vi "HEWH RLT PRAT.vi"() -> ()   [LabVIEW 2016] (continued)
        n1090 = Unbundle By Name(w2500) -> ("Plot Array C"=w2502:dbl[][], "C Data Array"=w2497:string[][], "File Locations C.New Summary Created"=w2498:bool, "Core HEWH Data Input C.LV Program"=w2491:T24)
        n1091 = case shown="\"PRAT\", \"HEWH RLT\"" w2491 {
          tunnel: [TRUE ("Reset After 24hrs") FALSE ("Reset After 24hrs")] -> w2490
          frame Default {
          }
          frame "PRAT", "HEWH RLT" {
          }
        }
        n1092 = Transpose 2D Array(2D array=w2497) -> (transposed array=w2496:string[][])
        n1093 = call <vilib>:"Add State(s) to Queue__jki_lib_state_machine.vi"("State(s) in (\"\")"=w2510) -> ("States Out"=w2509:string)  [unwired: 14 in]
        n1094 = call "UTILITY MultiPlot.vi"("Y-Axis-2"="Y-Axis2 - Station C", "Y-Axis-1"="Y-Axis1 - Station C", "X-Axis"="X-Axis - Station C", "Save Data"=w2496, "Plot Array"=w2502) -> ("Plot Cluster"=w2507:T34)  [unwired: 5 in, 1 out]
        n1095 = call "UTILITY Create Plot Array.vi"("Save Data"=w2496, "Plot Array in"=w2502) -> ("Plot Array out"=w2495:dbl[][])  [unwired: 8 in, 1 out]
        n1096 = call "UTILITY Array Reset.vi"("Reset After 24hrs"=w2490, "Plot Array Input"=w2495) -> ("Reset Array"=w2494:bool)  [unwired: 9 in]
        n1097 = case shown="False" "Pause Graph C" {
          tunnel: w2507 -> [w2517 _]
          tunnel: "X-Axis - Station C" -> [w2516 _]
          tunnel: "Y-Axis1 - Station C" -> [w2515 _]
          frame False {
            n1098 = property on="XY Graph - Station C" class="XYGraph (strict)"("XScale.NameLbl.Text"=w2516, "YScale.NameLbl.Text"=w2515) -> ()  [unwired: 2 in, 2 out]
            "XY Graph - Station C" <- w2517
          }
          frame True {
          }
        }
        n1099 = Compound Arithmetic op=OR("Clear Graph Data C", w2498, w2494) -> (w2503:bool)
        n1100 = case shown="False" w2503 {
          tunnel: w2495 -> [w2513 _]
          tunnel: [w2513 dbl[][] [] ("Plot Array out")] -> w2506
          frame False {
          }
          frame True {
          }
        }
        n1101 = Bundle By Name(cluster=w2500, "Plot Array C"=w2506) -> (w2499:T80)
      }
      frame "Show Data D" {
        n1102 = Unbundle By Name(w2530) -> ("Plot Array D"=w2528:dbl[][], "D Data Array"=w2526:string[][], "File Locations D.New Summary Created"=w2527:bool, "Core HEWH Data Input D.LV Program"=w2519:T24)
        n1103 = case shown="\"PRAT\", \"HEWH RLT\"" w2519 {
          tunnel: [TRUE ("Reset After 24hrs") FALSE ("Reset After 24hrs")] -> w2518
          frame Default {
          }
          frame "PRAT", "HEWH RLT" {
          }
        }
        n1104 = Transpose 2D Array(2D array=w2526) -> (transposed array=w2525:string[][])
        n1105 = call <vilib>:"Add State(s) to Queue__jki_lib_state_machine.vi"("State(s) in (\"\")"=w2538) -> ("States Out"=w2537:string)  [unwired: 14 in]
        n1106 = call "UTILITY MultiPlot.vi"("Y-Axis-2"="Y-Axis2 - Station D", "Y-Axis-1"="Y-Axis1 - Station D", "X-Axis"="X-Axis - Station D", "Save Data"=w2525, "Plot Array"=w2528) -> ("Plot Cluster"=w2535:T34)  [unwired: 5 in, 1 out]
        n1107 = call "UTILITY Create Plot Array.vi"("Save Data"=w2525, "Plot Array in"=w2528) -> ("Plot Array out"=w2524:dbl[][])  [unwired: 8 in, 1 out]
        n1108 = call "UTILITY Array Reset.vi"("Reset After 24hrs"=w2518, "Plot Array Input"=w2524) -> ("Reset Array"=w2523:bool)  [unwired: 9 in]
        n1109 = case shown="False" "Pause Graph D" {
          tunnel: w2535 -> [w2545 _]
          tunnel: "X-Axis - Station D" -> [w2544 _]
          tunnel: "Y-Axis1 - Station D" -> [w2543 _]
          frame False {
            n1110 = property on="XY Graph - Station D" class="XYGraph (strict)"("XScale.NameLbl.Text"=w2544, "YScale.NameLbl.Text"=w2543) -> ()  [unwired: 2 in, 2 out]
            "XY Graph - Station D" <- w2545
          }
          frame True {
          }
        }
        n1111 = Compound Arithmetic op=OR("Clear Graph Data D", w2527, w2523) -> (w2531:bool)
        n1112 = case shown="False" w2531 {
          tunnel: w2524 -> [w2541 _]
          tunnel: [w2541 dbl[][] [] ("Plot Array out")] -> w2534
          frame False {
          }
          frame True {
          }
        }
        n1113 = Bundle By Name(cluster=w2530, "Plot Array D"=w2534) -> (w2529:T80)
      }
      frame "Data: Save Data" {
        # "Probably better to pull the whole control in. Would just have to do some event sequencing...guess this is lazy"
        n1114 = local read "Appliance Details A"() -> (w2550:T4)
        n1115 = local read "Appliance Details B"() -> (w2549:T4)
        n1116 = local read "Appliance Details C"() -> (w2548:T4)
        n1117 = local read "Appliance Details D"() -> (w2547:T4)
        n1118 = Unbundle By Name(w2571) -> ("File Locations A"=w2566:T2, "File Locations B"=w2565:T2, "File Locations C"=w2564:T2, "File Locations D"=w2563:T2, "A Data Array"=w2562:string[][], "B Data Array"=w2561:string[][], "C Data Array"=w2560:string[][], "D Data Array"=w2559:string[][])
        n1119 = Build Array(w2550, w2549, w2548, w2547) -> (w2546:T4[])
        n1120 = local read "Log Data Output (D)"() -> (w2551:bool)
        n1121 = local read "Log Data Output (C)"() -> (w2552:bool)
        n1122 = local read "Log Data Output (B)"() -> (w2553:bool)
        n1123 = local read "Log Data Output (A)"() -> (w2554:bool)
        n1124 = call "Save File Four Stations.vi"("File Locations A in"=w2566, "File Locations B in"=w2565, "File Locations C in"=w2564, "File Locations D in"=w2563, "Save Data A"=w2554, "A Data Array"=w2562, "Save Data B"=w2553, "B Data Array"=w2561, "Save Data C"=w2552, "C Data Array"=w2560, "Save Data D"=w2551, "D Data Array"=w2559, "Appliance Details"=w2546) -> ("Saving A"=w2558:bool, "File Locations A out"=w2570:T2, "File Locations B out"=w2569:T2, "File Locations C out"=w2568:T2, "File Locations D out"=w2567:T2, "Saving B"=w2557:bool, "Saving C"=w2556:bool, "Saving D"=w2555:bool)  [unwired: 6 in, 1 out]
        n1125 = Bundle By Name(cluster=w2571, "File Locations A"=w2570, "File Locations B"=w2569, "File Locations C"=w2568, "File Locations D"=w2567) -> (w2572:T80)
        n1126 = property on="Saving Display" class="Bool (strict)"("Value"=w2558) -> ()  [unwired: 2 in, 2 out]
        n1127 = property on="Saving Display" class="Bool (strict)"("Value"=w2557) -> ()  [unwired: 2 in, 2 out]
        n1128 = property on="Saving Display" class="Bool (strict)"("Value"=w2556) -> ()  [unwired: 2 in, 2 out]
        n1129 = property on="Saving Display" class="Bool (strict)"("Value"=w2555) -> ()  [unwired: 2 in, 2 out]
        n1130 = call <vilib>:"Add State(s) to Queue__jki_lib_state_machine.vi"("State(s) in (\"\")"=w2575) -> ("States Out"=w2574:string)  [unwired: 14 in]
      }
      frame "Add Final Data A" {
        n1131 = Unbundle By Name(w2584) -> ("File Locations A.Data File Paths.Data File Path"=w2588:path, "Core HEWH Data Input A.Calc and Calibration.All Draw Stats"=w2587:string[][])
        "All Draw Stats" <- w2587
        n1132 = call "UTILITY String Notifier.vi"("Status"=UTILITY_Notifier."Set", "error in (no error)"=w2577, "Set Status"="Writing Final Headers...", "name (unnamed)"="MessageA") -> ("error out"=w2576:errorcluster)  [unwired: 6 in, 1 out]
        n1133 = call "Save File Add Summary Data.vi"("Data That Has Been\nCollecting"=w2588, "Error In"=w2576, "Use 2D String Summary"=TRUE, "Add Final RMC"=FALSE, "2D String Summary"=w2587) -> ("Error Out"=w2582:errorcluster)  [unwired: 14 in]
        n1134 = flat-sequence {
          tunnel: w2584 -> [w2599]
          tunnel: [w2598] -> w2583
          tunnel: w2582 -> [w2595]
          tunnel: [w2594] -> w2581
          frame #0 {
            w2591 = FALSE ("Value")
            # "Used in auto test portion.\nTired of tinkering with\nevents"
            n1135 = property on="Saving Display" class="Bool (strict)"("Value"=w2591) -> ()  [unwired: 2 in, 2 out]
            n1136 = local write "Final Headers A"(w2591) -> ()
            n1137 = Bundle By Name(cluster=w2599, "File Locations A.Data File Paths"=T3 {"Data File Path"=path "", "Debug File Path"=path "", "Bus Log Path"=path "", "Current"=path "", "Summary"=path ""} ("Data File Paths")) -> (w2598:T80)
            n1138 = call "UTILITY String Notifier.vi"("Status"=UTILITY_Notifier."Set", "error in (no error)"=w2595, "Set Status"="", "name (unnamed)"="MessageA") -> ("error out"=w2594:errorcluster)  [unwired: 6 in, 1 out]
          }
        }
        n1139 = call <vilib>:"Add State(s) to Queue__jki_lib_state_machine.vi"("State(s) in (\"\")"=w2590) -> ("States Out"=w2589:string)  [unwired: 14 in]
      }
      frame "Add Final Data B" {
        n1140 = Unbundle By Name(w2607) -> ("File Locations B.Data File Paths.Data File Path"=w2612:path, "Core HEWH Data Input B.Calc and Calibration.All Draw Stats"=w2611:string[][])
        n1141 = call "UTILITY String Notifier.vi"("Status"=UTILITY_Notifier."Set", "error in (no error)"=w2601, "Set Status"="Writing Final Headers...", "name (unnamed)"="MessageB") -> ("error out"=w2600:errorcluster)  [unwired: 6 in, 1 out]
        n1142 = call "Save File Add Summary Data.vi"("Data That Has Been\nCollecting"=w2612, "Error In"=w2600, "Use 2D String Summary"=TRUE, "Add Final RMC"=FALSE, "2D String Summary"=w2611) -> ("Error Out"=w2608:errorcluster)  [unwired: 14 in]
        n1143 = flat-sequence {
          tunnel: w2607 -> [w2623]
          tunnel: [w2622] -> w2606
          tunnel: w2608 -> [w2619]
          tunnel: [w2618] -> w2605
          frame #0 {
            w2615 = FALSE ("Value")
            n1144 = property on="Saving Display" class="Bool (strict)"("Value"=w2615) -> ()  [unwired: 2 in, 2 out]
            n1145 = local write "Final Headers B"(w2615) -> ()
            n1146 = Bundle By Name(cluster=w2623, "File Locations B.Data File Paths"=T3 {"Data File Path"=path "", "Debug File Path"=path "", "Bus Log Path"=path "", "Current"=path "", "Summary"=path ""} ("Data File Paths")) -> (w2622:T80)
            n1147 = call "UTILITY String Notifier.vi"("Status"=UTILITY_Notifier."Set", "error in (no error)"=w2619, "Set Status"="", "name (unnamed)"="MessageB") -> ("error out"=w2618:errorcluster)  [unwired: 6 in, 1 out]
          }
        }
        n1148 = call <vilib>:"Add State(s) to Queue__jki_lib_state_machine.vi"("State(s) in (\"\")"=w2614) -> ("States Out"=w2613:string)  [unwired: 14 in]
      }
      frame "Add Final Data C" {
        n1149 = Unbundle By Name(w2631) -> ("File Locations C.Data File Paths.Data File Path"=w2636:path, "Core HEWH Data Input C.Calc and Calibration.All Draw Stats"=w2635:string[][])
        n1150 = call "UTILITY String Notifier.vi"("Status"=UTILITY_Notifier."Set", "error in (no error)"=w2625, "Set Status"="Writing Final Headers...", "name (unnamed)"="MessageC") -> ("error out"=w2624:errorcluster)  [unwired: 6 in, 1 out]
        n1151 = call "Save File Add Summary Data.vi"("Data That Has Been\nCollecting"=w2636, "Error In"=w2624, "Use 2D String Summary"=TRUE, "Add Final RMC"=FALSE, "2D String Summary"=w2635) -> ("Error Out"=w2632:errorcluster)  [unwired: 14 in]
        n1152 = flat-sequence {
          tunnel: w2631 -> [w2647]
          tunnel: [w2646] -> w2630
          tunnel: w2632 -> [w2643]
          tunnel: [w2642] -> w2629
          frame #0 {
            w2639 = FALSE ("Value")
            n1153 = local write "Final Headers C"(w2639) -> ()
            n1154 = Bundle By Name(cluster=w2647, "File Locations C.Data File Paths"=T3 {"Data File Path"=path "", "Debug File Path"=path "", "Bus Log Path"=path "", "Current"=path "", "Summary"=path ""} ("Data File Paths")) -> (w2646:T80)
            n1155 = property on="Saving Display" class="Bool (strict)"("Value"=w2639) -> ()  [unwired: 2 in, 2 out]
            n1156 = call "UTILITY String Notifier.vi"("Status"=UTILITY_Notifier."Set", "error in (no error)"=w2643, "Set Status"="", "name (unnamed)"="MessageC") -> ("error out"=w2642:errorcluster)  [unwired: 6 in, 1 out]
          }
        }
        n1157 = call <vilib>:"Add State(s) to Queue__jki_lib_state_machine.vi"("State(s) in (\"\")"=w2638) -> ("States Out"=w2637:string)  [unwired: 14 in]
      }
      frame "Add Final Data D" {
        n1158 = Unbundle By Name(w2655) -> ("File Locations D.Data File Paths.Data File Path"=w2660:path, "Core HEWH Data Input D.Calc and Calibration.All Draw Stats"=w2659:string[][])
        n1159 = call "UTILITY String Notifier.vi"("Status"=UTILITY_Notifier."Set", "error in (no error)"=w2650, "Set Status"="Writing Final Headers...", "name (unnamed)"="MessageD") -> ("error out"=w2649:errorcluster)  [unwired: 6 in, 1 out]
        n1160 = call "Save File Add Summary Data.vi"("Data That Has Been\nCollecting"=w2660, "Error In"=w2649, "Use 2D String Summary"=TRUE, "Add Final RMC"=FALSE, "2D String Summary"=w2659) -> ("Error Out"=w2656:errorcluster)  [unwired: 14 in]
        n1161 = flat-sequence {
          tunnel: w2655 -> [w2671]
          tunnel: [w2670] -> w2654
          tunnel: w2656 -> [w2667]
          tunnel: [w2666] -> w2653
          frame #0 {
            w2663 = FALSE ("Value")
            n1162 = property on="Saving Display" class="Bool (strict)"("Value"=w2663) -> ()  [unwired: 2 in, 2 out]
            n1163 = local write "Final Headers D"(w2663) -> ()
            n1164 = Bundle By Name(cluster=w2671, "File Locations D.Data File Paths"=T3 {"Data File Path"=path "", "Debug File Path"=path "", "Bus Log Path"=path "", "Current"=path "", "Summary"=path ""} ("Data File Paths")) -> (w2670:T80)
            n1165 = call "UTILITY String Notifier.vi"("Status"=UTILITY_Notifier."Set", "error in (no error)"=w2667, "Set Status"="", "name (unnamed)"="MessageD") -> ("error out"=w2666:errorcluster)  [unwired: 6 in, 1 out]
          }
        }
        n1166 = call <vilib>:"Add State(s) to Queue__jki_lib_state_machine.vi"("State(s) in (\"\")"=w2662) -> ("States Out"=w2661:string)  [unwired: 14 in]
      }
      frame "-----Simple Processing-----" {
      }
      frame "Calculate Max AVG TC Temp" {
        n1167 = Unbundle By Name(w2675) -> ("Core HEWH Data Input A"=w2694:T12, "Core HEWH Data Input B"=w2692:T12, "Core HEWH Data Input C"=w2689:T12, "Core HEWH Data Input D"=w2688:T12)
        n1168 = local read "Current Draw Parameters"() -> (w2680:T41)
        n1169 = Unbundle By Name(w2680) -> ("Station A.Use Temp Decline Method"=w2679:bool, "Station B.Use Temp Decline Method"=w2678:bool, "Station C.Use Temp Decline Method"=w2677:bool, "Station D.Use Temp Decline Method"=w2676:bool)
        n1170 = case shown="True" w2679 {
          tunnel: w2694 -> [_ w2723]
          tunnel: [w2718 w2722] -> w2693
          tunnel: w2687 -> [w2718 w2721]
          tunnel: "Temperature Decline Amount (°F)" -> [_ w2720]
          tunnel: [TRUE ("Temp Decline Complete") w2719] -> w2684
          frame False {
          }
          frame True {
            n1171 = call "HEWH Determine When Too Draw.vi"("Last Draw TC Tree AVG Decline Amount (Degrees F)"=w2720, "Error In"=w2721, "Core HEWH Data IN"=w2723) -> ("Error Out"=w2722:errorcluster, "Temp Decline Complete"=w2719:bool)  [unwired: 7 in]
          }
        }
        "Temp Decline Complete A" <- w2684
        n1172 = case shown="False" w2678 {
          tunnel: w2693 -> [w2711 w2716]
          tunnel: w2692 -> [_ w2715]
          tunnel: [w2711 w2714] -> w2691
          tunnel: "Temperature Decline Amount (°F)" -> [_ w2713]
          tunnel: [TRUE ("Temp Decline Complete") w2712] -> w2683
          frame False {
          }
          frame True {
            n1173 = call "HEWH Determine When Too Draw.vi"("Last Draw TC Tree AVG Decline Amount (Degrees F)"=w2713, "Error In"=w2716, "Core HEWH Data IN"=w2715) -> ("Error Out"=w2714:errorcluster, "Temp Decline Complete"=w2712:bool)  [unwired: 7 in]
          }
        }
        "Temp Decline Complete B" <- w2683
        n1174 = case shown="True" w2677 {
          tunnel: w2691 -> [w2704 w2709]
          tunnel: [w2704 w2708] -> w2690
          tunnel: w2689 -> [_ w2707]
          tunnel: "Temperature Decline Amount (°F)" -> [_ w2706]
          tunnel: [TRUE ("Temp Decline Complete") w2705] -> w2682
          frame False {
          }
          frame True {
            n1175 = call "HEWH Determine When Too Draw.vi"("Last Draw TC Tree AVG Decline Amount (Degrees F)"=w2706, "Error In"=w2709, "Core HEWH Data IN"=w2707) -> ("Error Out"=w2708:errorcluster, "Temp Decline Complete"=w2705:bool)  [unwired: 7 in]
          }
        }
        "Temp Decline Complete C" <- w2682
        n1176 = case shown="True" w2676 {
          tunnel: w2690 -> [w2697 w2702]
          tunnel: w2688 -> [_ w2701]
          tunnel: [w2697 w2700] -> w2686
          tunnel: "Temperature Decline Amount (°F)" -> [_ w2699]
          tunnel: [TRUE ("Temp Decline Complete") w2698] -> w2681
          frame False {
          }
          frame True {
            n1177 = call "HEWH Determine When Too Draw.vi"("Last Draw TC Tree AVG Decline Amount (Degrees F)"=w2699, "Error In"=w2702, "Core HEWH Data IN"=w2701) -> ("Error Out"=w2700:errorcluster, "Temp Decline Complete"=w2698:bool)  [unwired: 7 in]
          }
        }
        "Temp Decline Complete D" <- w2681
      }
    }
    n1178 = local read "Debug"() -> (w1383:bool)
    n1179 = case shown="True" w1383 {
      tunnel: [w1397 w1400] -> w1382
      tunnel: w1385 -> [w1397 w1399]
      tunnel: w1384 -> [_ w1398]
      frame False {
      }
      frame True {
        n1180 = Build Array (concatenate)(w1399, w1398) -> (w1400:string[])
      }
    }
    "DAQ" <- w1382
  }
  n1181 = while {
    tunnel: w81 -> [w2733]
    tunnel: [w2742] -> _
    tunnel: w78 -> [w2741]
    tunnel: w116 -> [w2728]
    tunnel: w107 -> [w2729]
    tunnel: w67 -> [w2725]
    i -> [w2740]
    stop <- w2739 stop-if-true
    n1182 = local read "Finish"() -> (w2739:bool)
    n1183 = Dequeue Element(queue=w2728, error in (no error)=w2733) -> (element=w2730:T54, error out=w2732:errorcluster)  [unwired: 1 in, 2 out]
    n1184 = Unbundle By Name(w2730) -> ("Start Draw"=w2726:bool, "Station ID"=w2731:T25, "Station Draw Info"=w2727:T14, "Send Condition"=w2724:T1)
    "Start Draw" <- w2726
    n1185 = Wait Until Next ms Multiple(millisecond multiple=u32 100) -> ()  [unwired: 1 out]
    n1186 = case shown="\"A\", Default" w2731 {
      tunnel: [w2743 w2744 w2745 w2746] -> w2737
      frame "A", Default {
        n1187 = local read "Disable Station 1"() -> (w2743:T31)
      }
      frame "B" {
        n1188 = local read "Disable Station 2"() -> (w2744:T31)
      }
      frame "C" {
        n1189 = local read "Disable Station 3"() -> (w2745:T31)
      }
      frame "D" {
        n1190 = local read "Disable Station 4"() -> (w2746:T31)
      }
    }
    n1191 = Equal?(x=HEWH_RLT_Station_Disable."Enable Station", y=w2737) -> (x = y?=w2735:bool)
    n1192 = And(x=w2726, y=w2735) -> (x .and. y?=w2734:bool)
    n1193 = case shown="True" w2734 {
      tunnel: w2732 -> [w2747 w2771]
      tunnel: [w2747 w2770] -> w2742
      tunnel: w2741 -> [_ w2764]
      tunnel: w2731 -> [_ w2753]
      tunnel: w2729 -> [_ w2762]
      tunnel: w2727 -> [_ w2754]
      tunnel: w2725 -> [_ w2755]
      tunnel: w2724 -> [_ w2751]
      frame False {
      }
      frame True {
        # "This is everything required to draw water"
        n1194 = flat-sequence {
          tunnel: w2771 -> [w2860]
          tunnel: [w2860] -> w2769
          frame #0 {
            n1195 = local write "Draw Complete"(FALSE ("Draw Complete")) -> ()
            n1196 = property on="Scan Rate (Seconds)" class="DigNum (strict)"("Value"=T10 1.0 ("Scan Rate (Seconds)")) -> ()  [unwired: 2 in, 2 out]
          }
        }
        n1197 = local read "Pressurize Tank?"() -> (w2761:bool)
        n1198 = local read "Use Emerson 5700"() -> (w2748:bool)
        n1199 = local read "Yokogawa WT210"() -> (w2758:refnum<visa-resource-name>)
        n1200 = local read "K-Factor Intellifaucet"() -> (w2759:dbl)
        n1201 = local read "MW100"() -> (w2768:refnum<visa-resource-name>)
        n1202 = local read "Laurel Hot IP Address"() -> (w2750:string)
        n1203 = case shown="\"D\"" w2753 {
          tunnel: w2769 -> [w2789 w2807 w2825 w2843]
          tunnel: w2768 -> [w2788 w2804 w2824 w2842]
          tunnel: "Purge Time (Seconds)" -> [w2787 w2803 w2821 w2841]
          tunnel: [w2776 w2794 w2812 w2830] -> w2767
          tunnel: w2754 -> [w2786 w2802 w2814 w2840]
          tunnel: "Skip Purge" -> [w2784 w2805 w2823 w2839]
          tunnel: "Skip Draw" -> [w2783 w2806 w2822 w2838]
          tunnel: w2764 -> [w2785 w2799 w2819 w2837]
          tunnel: w2761 -> [w2780 w2798 w2818 w2834]
          tunnel: w2759 -> [w2779 w2797 w2817 w2833]
          tunnel: w2758 -> [w2777 w2795 w2815 w2831]
          tunnel: w2751 -> [w2774 w2792 w2810 w2828]
          tunnel: w2750 -> [w2773 w2791 w2809 w2827]
          tunnel: w2748 -> [w2772 w2790 w2808 w2826]
          frame "A", Default {
            n1204 = local read "Core HEWH Data Input A"() -> (w2782:T12)
            n1205 = local read "GEA2_A?"() -> (w2775:bool)
            n1206 = call "HEWH Purge Draw Sequence.vi"("MW100"=w2788, "Purge Time (Seconds)"=w2787, "Station Draw Info"=w2786, "Current Cond"=w2774, "Laurel Hot IP Address"=w2773, "Error In"=w2789, "Skip Purge"=w2784, "Core HEWH Data Input"=w2782, "Skip Draw"=w2783, "MW100 Sema"=w2785, "K-Factor (Intellifaucet)"=w2779, "Pressurize Tank?"=w2780, "Use Fuzzy Logic"=FALSE, "GEA2?"=w2775, "Yokogawa WT210"=w2777, "Use Emerson 5700?"=w2772) -> ("Core HEWH Data out"=→"Station A Update":T12, "Error Out"=w2776:errorcluster)  [unwired: 2 in]
          }
          frame "B" {
            n1207 = local read "Core HEWH Data Input B"() -> (w2801:T12)
            n1208 = local read "GEA2_B?"() -> (w2793:bool)
            n1209 = call "HEWH Purge Draw Sequence.vi"("MW100"=w2804, "Purge Time (Seconds)"=w2803, "Station Draw Info"=w2802, "Current Cond"=w2792, "Laurel Hot IP Address"=w2791, "Error In"=w2807, "Skip Purge"=w2805, "Core HEWH Data Input"=w2801, "Skip Draw"=w2806, "MW100 Sema"=w2799, "K-Factor (Intellifaucet)"=w2797, "Pressurize Tank?"=w2798, "Use Fuzzy Logic"=FALSE, "GEA2?"=w2793, "Yokogawa WT210"=w2795, "Use Emerson 5700?"=w2790) -> ("Core HEWH Data out"=→"Station B Update":T12, "Error Out"=w2794:errorcluster)  [unwired: 2 in]
          }
          frame "C" {
            n1210 = local read "Core HEWH Data Input C"() -> (w2813:T12)
            n1211 = local read "GEA2_C?"() -> (w2811:bool)
            n1212 = call "HEWH Purge Draw Sequence.vi"("MW100"=w2824, "Purge Time (Seconds)"=w2821, "Station Draw Info"=w2814, "Current Cond"=w2810, "Laurel Hot IP Address"=w2809, "Error In"=w2825, "Skip Purge"=w2823, "Core HEWH Data Input"=w2813, "Skip Draw"=w2822, "MW100 Sema"=w2819, "K-Factor (Intellifaucet)"=w2817, "Pressurize Tank?"=w2818, "Use Fuzzy Logic"=FALSE, "GEA2?"=w2811, "Yokogawa WT210"=w2815, "Use Emerson 5700?"=w2808) -> ("Core HEWH Data out"=→"Station C Update":T12, "Error Out"=w2812:errorcluster)  [unwired: 2 in]
          }
          frame "D" {
            n1213 = local read "Core HEWH Data Input D"() -> (w2836:T12)
            n1214 = local read "GEA2_D?"() -> (w2829:bool)
            n1215 = call "HEWH Purge Draw Sequence.vi"("MW100"=w2842, "Purge Time (Seconds)"=w2841, "Station Draw Info"=w2840, "Current Cond"=w2828, "Laurel Hot IP Address"=w2827, "Error In"=w2843, "Skip Purge"=w2839, "Core HEWH Data Input"=w2836, "Skip Draw"=w2838, "MW100 Sema"=w2837, "K-Factor (Intellifaucet)"=w2833, "Pressurize Tank?"=w2834, "Use Fuzzy Logic"=FALSE, "GEA2?"=w2829, "Yokogawa WT210"=w2831, "Use Emerson 5700?"=w2826) -> ("Core HEWH Data out"=→"Station D Update":T12, "Error Out"=w2830:errorcluster)  [unwired: 2 in]
          }
        }
        n1216 = flat-sequence {
          tunnel: [w2845] -> w2757
          tunnel: w2762 -> [w2847]
          tunnel: w2767 -> [w2846]
          tunnel: [w2844] -> w2756
          tunnel: w2757 -> [w2851]
          tunnel: [w2850] -> w2752
          tunnel: w2756 -> [w2849]
          tunnel: w2755 -> [w2848]
          tunnel: w2752 -> [w2853]
          tunnel: [w2853] -> w2760
          tunnel: w2760 -> [w2857]
          tunnel: [w2856] -> w2770
          tunnel: w2749 -> [w2854]
          frame #0 {
            w2844 = TRUE ("Draw Start")
            n1217 = Generate User Event(user event=w2847, event data cluster=w2844, error in=w2846) -> (error out=w2845:errorcluster)  [unwired: 1 in, 1 out]
            "Draw Complete" <- w2844
          }
          frame #1 {
            n1218 = Generate User Event(user event=w2848, event data cluster=w2849, error in=w2851) -> (error out=w2850:errorcluster)  [unwired: 1 in, 1 out]
          }
          frame #2 {
            n1219 = local write "Start Draw"(FALSE ("Start Draw")) -> ()
          }
          frame #3 {
            n1220 = property on="Scan Rate (Seconds)" class="DigNum (strict)"("Value"=w2854) -> ()  [unwired: 2 in, 2 out]
            n1221 = call "UTILITY Delay mS.vi"("Error In"=w2857, "milliseconds to wait"=u32 1000) -> ("Error Out"=w2856:errorcluster)  [unwired: 13 in]
          }
        }
        n1222 = local read "Scan Rate (Default)"() -> (w2749:T10)
      }
    }
    "Draw Loop" <- w2740
  }
  n1223 = while "UI Events" {
    shift-right: [w2879] -> _
    shift-left: _ -> [w2878]
    shift-right: [w2882] -> _
    shift-left: w25 -> [w2876]
    shift-right: [w2881] -> _
    shift-left: w126 -> [w2883]
    tunnel: w78 -> [w2875]
    tunnel: w24 -> [w2874]
    tunnel: w23 -> [w2873]
    tunnel: w51 -> [w2872]
    tunnel: w50 -> [w2871]
    tunnel: w49 -> [w2870]
    tunnel: w48 -> [w2869]
    tunnel: w45 -> [w2868]
    tunnel: w44 -> [w2867]
    tunnel: w43 -> [w2866]
    tunnel: w42 -> [w2865]
    tunnel: w41 -> [w2864]
    tunnel: w40 -> [w2863]
    tunnel: w39 -> [w2862]
    tunnel: w38 -> [w2861]
    stop <- w2880 stop-if-true
    w2877 = 500  # Timeout
    # "UI Events"
    n1224 = call <vilib>:"Parse State Queue__JKI_lib_State_Machine.vi"("State Queue"=w2883, "Error In (no error)"=w2876) -> ("Remaining States"=w2885:string, "Current State"=w2886:string, "Arguments"=w2884:string)  [unwired: 11 in]
    "UI State" <- w2886
    n1225 = case shown="\"\", \"Idle\"" w2886 {
      selector: w2886 -> [_ _ w3495 _ _ _ _ _ _ _ _ _ _ _ _ _ _ _ _ _ _ _ _ _ _ _ _ _ _ _ _ _ _ _ _]
      tunnel: w2885 -> [w2908 w3494 w3499 w3511 w3516 w3520 w3534 w3550 w3554 w3559 w3571 w3593 w3615 w3637 w3659 w3671 w3683 w3695 w3707 w3719 w3731 w3743 w3758 w3764 w3779 w3800 w3810 w3820 w3831 w3839 w3840 w3845 w3883 w3928 w3945]
      tunnel: w2884 -> [_ _ _ _ _ _ _ _ _ _ _ _ _ _ _ _ _ _ _ _ _ _ _ _ _ _ _ _ _ _ _ _ _ _ _]
      tunnel: w2878 -> [w2906 w3491 w3497 w3508 w3514 w3517 _ w3547 w3551 w3556 w3569 w3591 w3613 w3635 w3657 w3669 w3681 w3693 w3705 w3717 w3729 w3741 w3755 w3761 w3773 w3797 w3805 w3815 w3829 w3833 w3841 w3850 w3884 w3927 w3943]
      tunnel: [w2905 w3492 w3501 errorcluster {"status"=FALSE, "code"=0, "source"=""} ("error out") w3513 w3518 w3532 w3548 w3552 w3557 w3566 w3588 w3610 w3632 w3652 w3662 w3674 w3685 w3699 w3710 w3723 w3734 w3750 w3762 w3772 w3791 w3804 w3814 w3826 w3834 w3842 w3851 w3885 w3929 w3944] -> w2882
      tunnel: w2876 -> [w2904 w3492 w3500 w3507 w3513 w3518 w3532 w3548 w3552 w3557 w3568 w3590 w3612 w3634 w3655 w3666 w3678 w3690 w3703 w3714 w3726 w3738 w3754 w3762 w3769 w3787 w3803 w3813 w3827 w3835 w3842 w3851 w3885 w3929 w3944]
      tunnel: [w2907 w3493 w3498 w3510 w3515 w3519 w3533 w3549 w3553 w3558 w3570 w3592 w3614 w3636 w3658 w3670 w3682 w3694 w3706 w3718 w3730 w3742 w3757 w3763 w3778 w3799 w3809 w3819 w3830 w3838 w3840 w3844 w3881 w3926 w3945] -> w2881
      tunnel: [_ _ _ _ TRUE _ _ _ _ _ _ _ _ _ _ _ _ _ _ _ _ _ _ _ _ _ _ _ _ _ _ _ _ _ _] -> w2880
      tunnel: [w2903 w3491 w3497 w3508 w3514 w3517 w3526 w3547 w3551 w3556 w3569 w3591 w3613 w3635 w3657 w3669 w3681 w3693 w3705 w3717 w3729 w3741 w3755 w3761 w3773 w3797 w3805 w3815 w3829 w3833 w3841 w3843 w3882 w3927 w3942] -> w2879
      tunnel: w2877 -> [w2902 _ _ _ _ _ _ _ _ _ _ _ _ _ _ _ _ _ _ _ _ _ _ _ _ _ _ _ _ _ _ _ _ _ _]
      tunnel: w2875 -> [w2899 _ _ _ _ _ _ _ _ _ w3567 w3589 w3611 w3633 w3650 w3664 w3676 w3688 w3701 w3713 w3722 w3737 w3752 _ w3767 w3785 w3802 w3812 w3825 w3832 _ _ _ _ _]
      tunnel: w2874 -> [w2901 _ _ _ _ _ _ _ _ _ _ _ _ _ _ _ _ _ _ _ _ _ _ _ _ _ _ _ _ _ _ _ _ _ _]
      tunnel: w2873 -> [w2900 _ _ _ _ _ _ _ _ _ _ _ _ _ _ _ _ _ _ _ _ _ _ _ _ _ _ _ _ _ _ _ _ _ _]
      tunnel: w2872 -> [w2898 _ _ _ _ _ _ _ _ _ _ _ _ _ _ _ _ _ _ _ _ _ _ _ _ _ _ _ _ _ _ _ _ _ _]
      tunnel: w2871 -> [w2897 _ _ _ _ _ _ _ _ _ _ _ _ _ _ _ _ _ _ _ _ _ _ _ _ _ _ _ _ _ _ _ _ _ _]
      tunnel: w2870 -> [w2896 _ _ _ _ _ _ _ _ _ _ _ _ _ _ _ _ _ _ _ _ _ _ _ _ _ _ _ _ _ _ _ _ _ _]
      tunnel: w2869 -> [w2895 _ _ _ _ _ _ _ _ _ _ _ _ _ _ _ _ _ _ _ _ _ _ _ _ _ _ _ _ _ _ _ _ _ _]
      tunnel: w2868 -> [w2894 _ _ _ _ _ _ _ _ _ _ _ _ _ _ _ _ _ _ _ _ _ _ _ _ _ _ _ _ _ _ _ _ _ _]
      tunnel: w2867 -> [w2893 _ _ _ _ _ _ _ _ _ _ _ _ _ _ _ _ _ _ _ _ _ _ _ _ _ _ _ _ _ _ _ _ _ _]
      tunnel: w2866 -> [w2892 _ _ _ _ _ _ _ _ _ _ _ _ _ _ _ _ _ _ _ _ _ _ _ _ _ _ _ _ _ _ _ _ _ _]
      tunnel: w2865 -> [w2891 _ _ _ _ _ _ _ _ _ _ _ _ _ _ _ _ _ _ _ _ _ _ _ _ _ _ _ _ _ _ _ _ _ _]
      tunnel: w2864 -> [w2890 _ _ _ _ _ _ _ _ _ _ _ _ _ _ _ _ _ _ _ _ _ _ _ _ _ _ _ _ _ _ _ _ _ _]
      tunnel: w2863 -> [w2889 _ _ _ _ _ _ _ _ _ _ _ _ _ _ _ _ _ _ _ _ _ _ _ _ _ _ _ _ _ _ _ _ _ _]
      tunnel: w2862 -> [w2888 _ _ _ _ _ _ _ _ _ _ _ _ _ _ _ _ _ _ _ _ _ _ _ _ _ _ _ _ _ _ _ _ _ _]
      tunnel: w2861 -> [w2887 _ _ _ _ _ _ _ _ _ _ _ _ _ _ _ _ _ _ _ _ _ _ _ _ _ _ _ _ _ _ _ _ _ _]
      frame "", "Idle" {
        n1226 = event shown="[3] \"Reset Inventory\": Value Change" {
          selector: _ -> [_ _ _ _ _ _ _ _ _ _ _ _ _ _ _ _ _ _ _ _ _ _ _ _ _ _ _ _ _ _ _ _ _ _ _ _ _ _ _ _ _]
          dyn-events: _ -> [_ _ _ _ _ _ _ _ _ _ _ _ _ _ _ _ _ _ _ _ _ _ _ _ _ _ _ _ _ _ _ _ _ _ _ _ _ _ _ _ _]
          timeout: w2902 -> [_ _ _ _ _ _ _ _ _ _ _ _ _ _ _ _ _ _ _ _ _ _ _ _ _ _ _ _ _ _ _ _ _ _ _ _ _ _ _ _ _]
          tunnel: w2908 -> [w2914 w2919 w2932 w2937 w2939 w2952 w2957 w2965 w2972 w2978 w2985 w2992 w2999 w3006 w3014 w3021 w3028 w3035 w3041 w3048 w3055 w3062 w3067 w3099 w3146 w3191 w3236 w3257 w3264 w3271 w3277 w3285 w3318 w3414 w3425 w3435 w3447 w3452 w3473 w3480 w3490]
          tunnel: [w2913 w2920 w2932 w2937 w2939 w2951 w2956 w2966 w2971 w2979 w2986 w2993 w3000 w3007 w3015 w3022 w3029 w3036 w3042 w3049 w3056 w3063 w3066 w3099 w3146 w3191 w3236 w3257 w3264 w3271 w3277 w3285 w3318 w3414 w3425 w3435 w3447 w3452 w3474 w3481 w3489] -> w2907
          tunnel: w2906 -> [w2910 w2921 w2925 w2938 w2940 w2953 w2958 w2961 w2968 w2976 w2983 w2990 w2997 w3003 w3011 w3018 w3025 w3032 w3039 w3045 w3052 w3059 w3069 w3100 w3147 w3192 w3237 w3258 w3265 w3272 w3278 w3286 w3319 w3415 w3426 w3436 w3448 w3453 w3472 w3478 w3487]
          tunnel: [w2912 w2917 w2930 w2934 w2941 w2954 w2959 w2963 w2973 w2980 w2987 w2994 w3001 w3008 w3009 w3016 w3023 w3030 w3043 w3050 w3057 w3064 w3065 w3093 w3139 w3185 w3230 w3256 w3263 w3270 w3279 w3290 w3310 w3413 w3424 w3437 w3446 w3450 w3469 w3479 w3488] -> w2905
          tunnel: w2904 -> [w2912 w2917 w2931 w2935 w2942 w2954 w2959 w2963 w2973 w2980 w2987 w2994 w3001 w3008 w3009 w3016 w3023 w3030 w3043 w3050 w3057 w3064 w3065 w3097 w3145 w3190 w3235 w3256 w3263 w3270 w3279 w3291 w3313 w3413 w3424 w3437 w3446 w3451 w3469 w3479 w3488]
          tunnel: [w2910 w2921 w2924 w2938 w2940 w2953 w2958 w2960 w2967 w2975 w2982 w2989 w2996 w3002 w3012 w3019 w3026 w3033 w3038 w3044 w3051 w3058 w3069 w3100 w3147 w3192 w3237 w3258 w3265 w3272 w3278 w3286 w3319 w3415 w3426 w3436 w3448 w3453 w3471 w3477 w3487] -> w2903
          tunnel: w2901 -> [_ _ _ _ _ _ _ _ _ _ _ _ _ _ _ _ _ _ _ _ _ _ _ w3092 w3138 w3184 w3228 _ _ _ _ _ _ _ _ _ _ _ _ _ _]
          tunnel: w2900 -> [_ _ _ _ _ _ _ _ _ _ _ _ _ _ _ _ _ _ _ _ _ _ _ w3087 w3134 w3179 w3224 _ _ _ _ _ _ _ _ _ _ _ _ _ _]
          tunnel: w2899 -> [_ _ w2929 _ _ _ _ _ _ _ _ _ _ _ _ _ _ _ _ _ _ _ _ _ _ _ _ _ _ _ _ w3288 _ _ _ _ _ _ _ _ _]
          tunnel: w2898 -> [_ _ _ _ _ _ _ _ _ _ _ _ _ _ _ _ _ _ _ _ _ _ _ w3076 _ _ _ _ _ _ _ _ _ _ _ _ _ _ _ _ _]
          tunnel: w2897 -> [_ _ _ _ _ _ _ _ _ _ _ _ _ _ _ _ _ _ _ _ _ _ _ _ w3121 _ _ _ _ _ _ _ _ _ _ _ _ _ _ _ _]
          tunnel: w2896 -> [_ _ _ _ _ _ _ _ _ _ _ _ _ _ _ _ _ _ _ _ _ _ _ _ _ w3167 _ _ _ _ _ _ _ _ _ _ _ _ _ _ _]
          tunnel: w2895 -> [_ _ _ _ _ _ _ _ _ _ _ _ _ _ _ _ _ _ _ _ _ _ _ _ _ _ w3212 _ _ _ _ _ _ _ _ _ _ _ _ _ _]
          tunnel: w2894 -> [_ _ _ _ _ _ _ _ _ _ _ _ _ _ _ _ _ _ _ _ _ _ _ _ _ _ _ _ _ _ _ _ w3301 _ _ _ _ _ _ _ _]
          tunnel: w2893 -> [_ _ _ _ _ _ _ _ _ _ _ _ _ _ _ _ _ _ _ _ _ _ _ _ _ _ _ _ _ _ _ _ w3303 _ _ _ _ _ _ _ _]
          tunnel: w2892 -> [_ _ _ _ _ _ _ _ _ _ _ _ _ _ _ _ _ _ _ _ _ _ _ _ _ _ _ _ _ _ _ _ w3305 _ _ _ _ _ _ _ _]
          tunnel: w2891 -> [_ _ _ _ _ _ _ _ _ _ _ _ _ _ _ _ _ _ _ _ _ _ _ _ _ _ _ _ _ _ _ _ w3307 _ _ _ _ _ _ _ _]
          tunnel: w2890 -> [_ _ _ _ _ _ _ _ _ _ _ _ _ _ _ _ _ _ _ _ _ _ _ _ _ _ _ _ _ _ _ _ w3308 _ _ _ _ _ _ _ _]
          tunnel: w2889 -> [_ _ _ _ _ _ _ _ _ _ _ _ _ _ _ _ _ _ _ _ _ _ _ _ _ _ _ _ _ _ _ _ w3306 _ _ _ _ _ _ _ _]
          tunnel: w2888 -> [_ _ _ _ _ _ _ _ _ _ _ _ _ _ _ _ _ _ _ _ _ _ _ _ _ _ _ _ _ _ _ _ w3304 _ _ _ _ _ _ _ _]
          tunnel: w2887 -> [_ _ _ _ _ _ _ _ _ _ _ _ _ _ _ _ _ _ _ _ _ _ _ _ _ _ _ _ _ _ _ _ w3302 _ _ _ _ _ _ _ _]
          event Timeout {
            n1227 = event-data() -> ()  [unwired: 1 in, 1 out]
            n1228 = Unbundle By Name(w2910) -> ("Hold Valves A"=w2909:bool)
            n1229 = case shown="True" w2909 {
              tunnel: ["" ("State(s) in Front (\"\")") "Hold Intellifaucet" ("State(s) in Front (\"\")")] -> w2911
              frame False {
              }
              frame True {
              }
            }
            n1230 = call <vilib>:"Add State(s) to Queue__jki_lib_state_machine.vi"("State(s) in Front (\"\")"=w2911, "State(s) in (\"\")"=w2914) -> ("States Out"=w2913:string)  [unwired: 13 in]
          }
          event "Finish": Value Change {
            n1231 = event-data() -> ()  [unwired: 1 in, 6 out]
            n1232 = call <vilib>:"Add State(s) to Queue__jki_lib_state_machine.vi"("State(s) in Front (\"\")"="Exit" ("State(s) in Front (\"\")"), "State(s) in (\"\")"=w2919) -> ("States Out"=w2920:string)  [unwired: 13 in]
          }
          event "Reset Flow Meter": Value Change {
            n1233 = event-data() -> ()  [unwired: 1 in, 6 out]
            n1234 = local read "Laurel Hot IP Address"() -> (w2928:string)
            n1235 = local read "Use Emerson 5700"() -> (w2922:bool)
            n1236 = Unbundle By Name(w2925) -> ("Test Fixture Hardware.Analog Data.Yokogawa.MW100"=w2927:refnum<visa-resource-name>)
            n1237 = call "HEWH Reset Flow Meter.vi"("Refnum in"=w2929, "Use Emerson 5700"=w2922, "error in (no error)"=w2931, "Debug"=FALSE, "Laurel Hot IP Address"=w2928, "dup VISA session in"=w2927) -> ("error out"=w2930:errorcluster, "VISA Refnum out"=w2923:refnum<visa-resource-name>)  [unwired: 4 in]
            n1238 = Bundle By Name(cluster=w2925, "Test Fixture Hardware.Analog Data.Yokogawa.MW100"=w2923) -> (w2924:T86)
          }
          event "Reset Inventory": Value Change {
            w2933 = T82 4 items=["Start/Stop Inventory 1"=367, "Start/Stop Inventory 2"=368, "Start/Stop all Totalizers and Inventories"=2, "Reset all Totalizers"=3, "Reset all Inventories"=4, "Reset Totalizer 1"=56, "Reset Totalizer 2"=57] ("Reset all Totalizers. 2")
            n1239 = event-data() -> ()  [unwired: 1 in, 6 out]
            n1240 = local read "Laurel Hot IP Address"() -> (w2936:string)
            n1241 = call "Emerson 5700 Reset Totalizers.vi"("Reset all Totalizers. 2"=w2933, "Error In"=w2935, "address"=w2936) -> ("Error Out"=w2934:errorcluster)  [unwired: 8 in]
          }
          event "Cancel Draw": Value Change {
            n1242 = event-data() -> ()  [unwired: 1 in, 6 out]
            n1243 = for {
              N: 10 -> [_]
              shift-right: [w2945] -> w2941
              shift-left: w2942 -> [w2946]
              n1244 = call "UTILITY Boolean Notifier.vi"("Status"=UTILITY_Notifier."Set", "error in (no error)"=w2946, "Set Status"=TRUE, "name (unnamed)"="Stop Custom Draw") -> ("error out"=w2945:errorcluster)  [unwired: 6 in, 1 out]
              n1245 = Wait Until Next ms Multiple(millisecond multiple=u32 10) -> ()  [unwired: 1 out]
            }
          }
          event "IF Start": Value Change {
            n1246 = event-data() -> ()  [unwired: 1 in, 6 out]
            n1247 = call <vilib>:"Add State(s) to Queue__jki_lib_state_machine.vi"("State(s) in Front (\"\")"="Start Intellifaucet\nAdjust Flow\nAdjust Temp" ("State(s) in Front (\"\")"), "State(s) in (\"\")"=w2952) -> ("States Out"=w2951:string)  [unwired: 13 in]
          }
          event "IF Stop": Value Change {
            n1248 = event-data() -> ()  [unwired: 1 in, 6 out]
            n1249 = call <vilib>:"Add State(s) to Queue__jki_lib_state_machine.vi"("State(s) in Front (\"\")"="Stop Intellifaucet\n" ("State(s) in Front (\"\")"), "State(s) in (\"\")"=w2957) -> ("States Out"=w2956:string)  [unwired: 13 in]
          }
          event "Valve % Open": Value Change {
            n1250 = event-data() -> ("NewVal"=w2962:dbl)  [unwired: 1 in, 5 out]
            n1251 = Bundle By Name(cluster=w2961, "User Controls.Percent Flow"=w2962) -> (w2960:T86)
            n1252 = call <vilib>:"Add State(s) to Queue__jki_lib_state_machine.vi"("State(s) in Front (\"\")"="Adjust Flow" ("State(s) in Front (\"\")"), "State(s) in (\"\")"=w2965) -> ("States Out"=w2966:string)  [unwired: 13 in]
          }
          event "Temp (°F)": Value Change {
            n1253 = event-data() -> ("NewVal"=w2969:dbl)  [unwired: 1 in, 5 out]
            n1254 = Bundle By Name(cluster=w2968, "User Controls.Intellifaucet \nTemperature"=w2969) -> (w2967:T86)
            n1255 = call <vilib>:"Add State(s) to Queue__jki_lib_state_machine.vi"("State(s) in Front (\"\")"="Adjust Temp", "State(s) in (\"\")"=w2972) -> ("States Out"=w2971:string)  [unwired: 13 in]
          }
          event "HEWH Power": Value Change {
            n1256 = event-data() -> ("NewVal"=w2974:bool)  [unwired: 1 in, 5 out]
            n1257 = Bundle By Name(cluster=w2976, "User Controls.Main Power Control"=w2974) -> (w2975:T86)
            n1258 = call <vilib>:"Add State(s) to Queue__jki_lib_state_machine.vi"("State(s) in Front (\"\")"="Main Power" ("State(s) in Front (\"\")"), "State(s) in (\"\")"=w2978) -> ("States Out"=w2979:string)  [unwired: 13 in]
          }
          event Value Change {
            n1259 = event-data() -> ("NewVal"=w2981:T37)  [unwired: 1 in, 5 out]
            n1260 = Bundle By Name(cluster=w2983, "User Controls.Valve Ctrl.Inlet Valve A"=w2981) -> (w2982:T86)
            n1261 = call <vilib>:"Add State(s) to Queue__jki_lib_state_machine.vi"("State(s) in Front (\"\")"="Inlet Valve A" ("State(s) in Front (\"\")"), "State(s) in (\"\")"=w2985) -> ("States Out"=w2986:string)  [unwired: 13 in]
          }
          event Value Change {
            n1262 = event-data() -> ("NewVal"=w2988:T37)  [unwired: 1 in, 5 out]
